vi "Test No Error When Project Contain Interface.vi"(8 "error in (no error)":errorcluster, 11 "Finder Test in":refnum<class "Finder Test.lvclass">) -> (0 "error out":errorcluster, 3 "Finder Test out":refnum<class "Finder Test.lvclass">)   [LabVIEW 2020, in "LUnit Tests.lvlib" / "Finder Test.lvclass"]
uses:
  Finder Test.lvclass
  C:/Program Files (x86)/National Instruments/LabVIEW 2020/vi.lib/Astemes/LUnit/Test Case.lvclass
  Finder Test.lvclass/Finder Test.ctl
  <vilib>/Astemes/LUnit/Test Case.lvclass/Test Case.ctl
  <vilib>/Astemes/LUnit/Palette/Pass.vi
  <vilib>/Astemes/LUnit/Palette/Fail.vi
  <vilib>/Astemes/LUnit/Set Assertion Type.vi
  <vilib>/Astemes/LUnit/Add test result.vi
  <vilib>/Astemes/LUnit/LUnit Record Assertion Result.vi
  <vilib>/Astemes/LUnit/LUnit Aggregate Assertion Results.vi
  <vilib>/Astemes/LUnit/Method Result/LUnit Merge Status.vi
  <vilib>/Astemes/LUnit/LUnit Concatenate result strings.vi
  source/Framework/Helper Classes/Test Finder/Test Finder.lvclass
  <vilib>/Astemes/LUnit/Test Case.lvclass
panel:
  out "error out 2":errorcluster
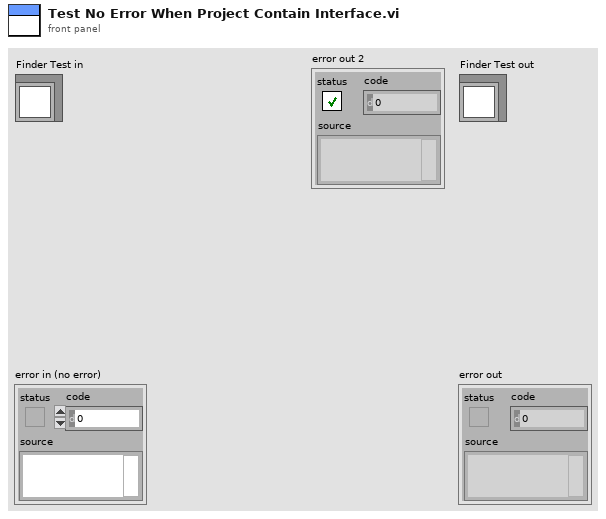
[diagram p1: front panel]
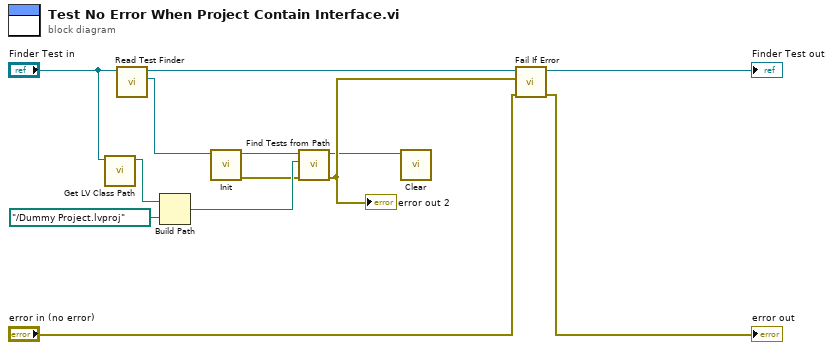
[diagram p0: block diagram]
diagram:
  n1 = call <vilib>:"Get LV Class Path.vi"("object"="Finder Test in") -> ("class path"=w10:path)  [unwired: 9 in, 1 out]
  n2 = call "Read Test Finder.vi"("Test Finder In"="Finder Test in") -> ("Test Finder.lvclass"=w3:refnum<class "Test Finder.lvclass">, "Test Finder Out"=w9:refnum<class "Finder Test.lvclass">)  [unwired: 8 in, 1 out]
  n3 = Build Path(base path=w10, name or relative path=path "../Dummy Project.lvproj") -> (appended path=w11:path)
  n4 = call-dynamic "Init.vi"("Test Finder in"=w3) -> ("error out"=w1:errorcluster, "Test Finder out"=w2:refnum<class "Test Finder.lvclass">)  [unwired: 9 in]
  n5 = call-dynamic "Find Tests from Path.vi"("error in (no error)"=w1, "Project or Class Path"=w11, "Test Case Finder In"=w2) -> ("error out"=w5:errorcluster, "Test Case Finder Out"=w4:refnum<class "Test Finder.lvclass">)  [unwired: 7 in]
  "error out 2" <- w5
  n6 = call "Clear.vi"("Test Finder in"=w4) -> ()  [unwired: 9 in, 2 out]
  n7 = call <vilib>:"Fail If Error.vi"("error in (no error)"="error in (no error)", "Assert error"=w5, "LUnit Test Case In"=w9) -> ("error out"=→"error out":errorcluster, "LUnit Test Case Out"=→"Finder Test out":refnum<class "Finder Test.lvclass">)  [unwired: 7 in]
